vi "GUI Init - DOM7.vi"(8 "error in (no error)":errorcluster, 9 "Ch.names":string[](array[string]), 10 "Cluster":T2, 11 "GUI Refs":T1) -> (0 "error out":errorcluster, 2 "Data":dbl[](array[numeric]), 3 "reference out":refnum<vi>)   [LabVIEW 2017]
doc: "Initialize array's size and values for DOM7 Array by reference"
uses:
  Controls/Discrete_GUI_Cluster.ctl
  Controls/GUI Referencies.ctl
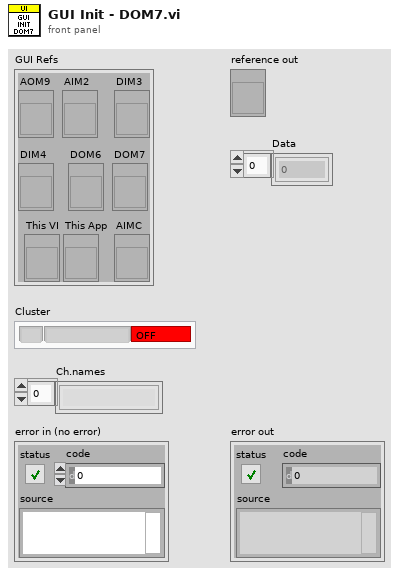
[diagram p1: front panel]
types:
  T1 = typedef "GUI Referencies.ctl" = cluster{"This VI":refnum<vi>, "This App":refnum<vi>, "DIM3":refnum<vi>, "DIM4":refnum<vi>, "DOM6":refnum<vi>, "DOM7":refnum<vi>, "AOM9":refnum<vi>, "AIM2":refnum<vi>, "AIMC":refnum<vi>}
  T2 = typedef "Discrete_GUI_Cluster.ctl" = cluster{"Ch.name":string, "Ch.state":bool, "Num":string}
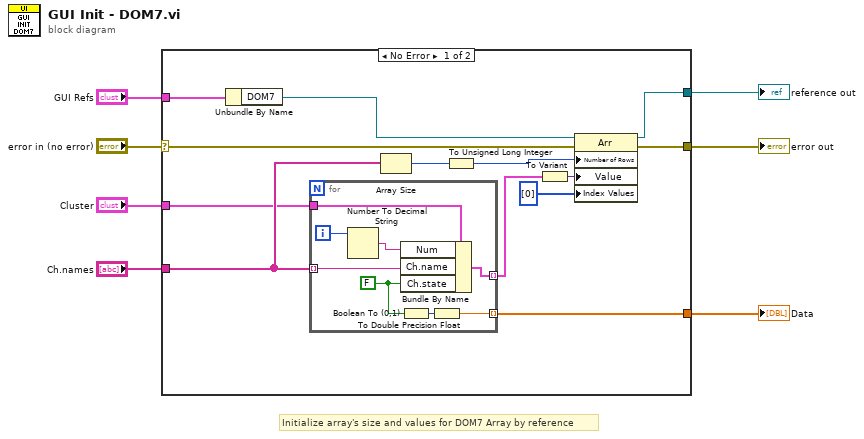
[diagram p0: block diagram]
diagram:
  # "Initialize array's size and values for DOM7 Array by reference"
  n1 = case shown="No Error" "error in (no error)" {
    selector: "error in (no error)" -> [w14 w29]
    tunnel: [w13 w29] -> w6
    tunnel: "Ch.names" -> [w17 _]
    tunnel: "GUI Refs" -> [w16 _]
    tunnel: "Cluster" -> [w15 _]
    tunnel: [w12 _] -> w3
    tunnel: [w8 _] -> w1
    frame No Error {
      n2 = Unbundle By Name(w16) -> ("DOM7"=w9:refnum<vi>)
      n3 = for {
        tunnel: [w28] -> w11 mode=indexing
        tunnel: w17 -> [w27] mode=indexing
        tunnel: w15 -> [w26]
        tunnel: [w23] -> w12 mode=indexing
        i -> [w22]
        w24 = FALSE
        n4 = Number To Decimal String(number=w22) -> (decimal integer string=w21:string)  [unwired: 1 in]
        n5 = Bundle By Name(cluster=w26, "Num"=w21, "Ch.name"=w27, "Ch.state"=w24) -> (w28:T2)
        n6 = Boolean To (0,1)(Boolean=w24) -> (0, 1=w25:i16)
        n7 = To Double Precision Float(number=w25) -> (double precision float=w23:dbl)
      }
      n8 = Array Size(array=w17) -> (size(s)=w19:i32)
      n9 = To Unsigned Long Integer(number=w19) -> (unsigned 32bit integer=w18:u32)
      n10 = To Variant(anything=w11) -> (Variant=w10:variant)
      n11 = property class="Arr"(reference=w9, error in=w14, "Number of Rows"=w18, "Value"=w10, "Index Values"=u32[] [0]) -> (reference out=w8:refnum<vi>, error out=w13:errorcluster)
    }
    frame Error {
    }
  }
  "error out" <- w6
  "Data" <- w3
  "reference out" <- w1
